vi "Get Station Number.vi"(8 "error in (no error)":errorcluster, 11 "UI Data in":T1) -> (0 "error out (no error)":errorcluster, 3 "UI Data out":T1)   [LabVIEW 2016]
uses:
  controls/GLDL UI Data.ctl
  controls/Disconnect Control.ctl
  controls/Download Control.ctl
  controls/Exit Control.ctl
  controls/Date Control.ctl
  controls/Save Path Control.ctl
  controls/COM Port Control.ctl
  controls/IP Phone Number Control.ctl
  controls/Connected Indicator.ctl
  controls/Output Indicator.ctl
  Message Queue/All Message Queues.ctl
  Message Queue/Message Cluster.ctl
  Message Queue/GLDL Message Queue.lvlib
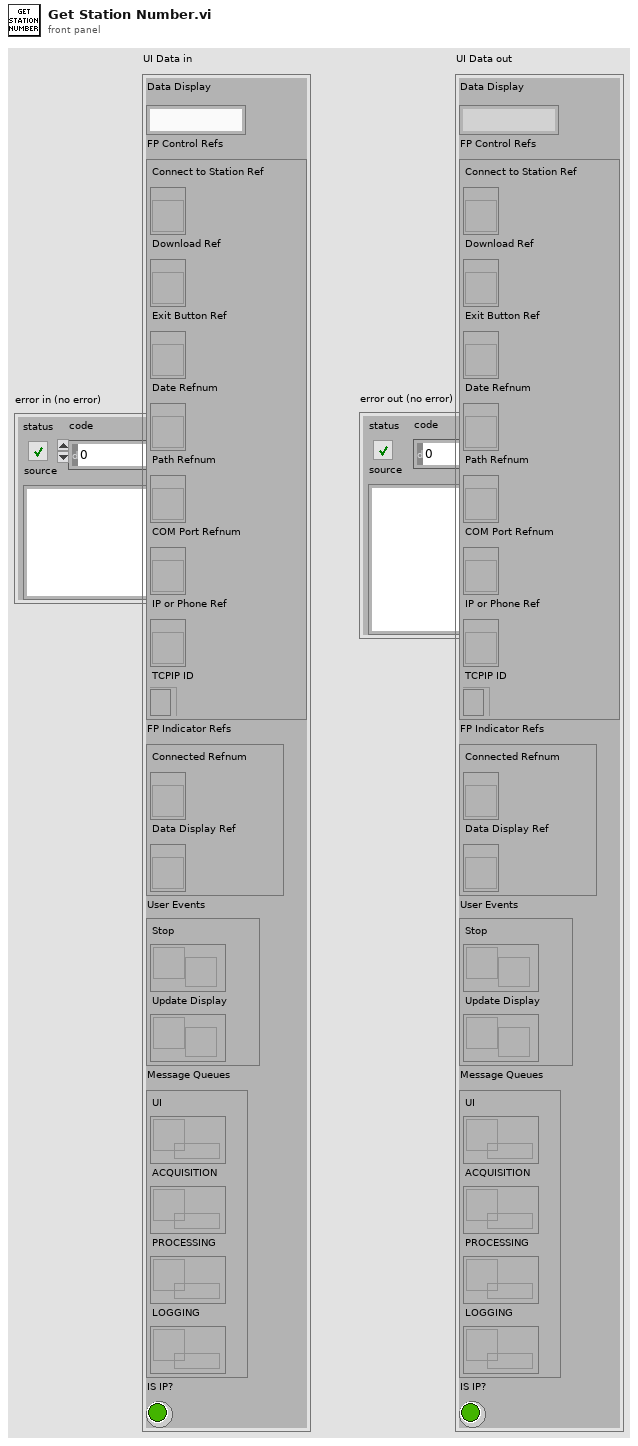
[diagram p1: front panel]
types:
  T1 = typedef "GLDL UI Data.ctl" = cluster{"Data Display":string, "FP Control Refs":cluster{"Connect to Station Ref":refnum<vi>, "Download Ref":refnum<vi>, "Exit Button Ref":refnum<vi>, "Date Refnum":refnum<vi>, "Path Refnum":refnum<vi>, "COM Port Refnum":refnum<vi>, "IP or Phone Ref":refnum<vi>, "TCPIP ID":refnum<k5>}, "FP Indicator Refs":cluster{"Connected Refnum":refnum<vi>, "Data Display Ref":refnum<vi>}, "User Events":cluster{"Stop":refnum<user-event>, "Update Display":refnum<user-event>}, "Message Queues":T2, "IS IP?":bool}
  T2 = typedef "GLDL Message Queue.lvlib/All Message Queues.ctl" = cluster{"UI":refnum<queue>, "ACQUISITION":refnum<queue>, "PROCESSING":refnum<queue>, "LOGGING":refnum<queue>}
  T3 = enum16{"Standard", "Buffered", "CRLF", "Immediate"}
  T4 = typedef "COM Port Control.ctl" = refnum<visa-resource-name>
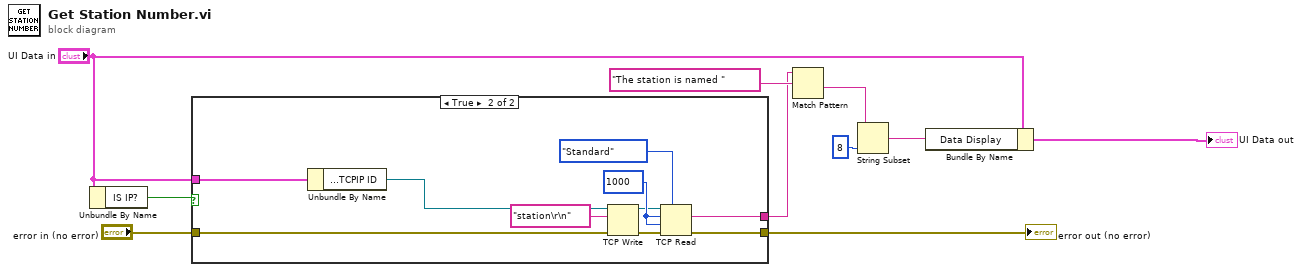
[diagram p0: block diagram]
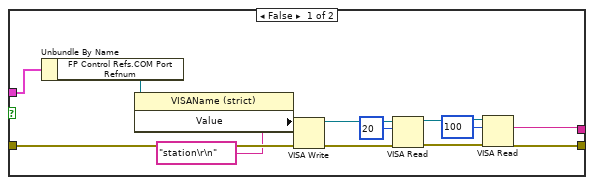
[diagram p2: hidden frame]
diagram:
  n1 = Unbundle By Name("UI Data in") -> ("IS IP?"=w3:bool)
  n2 = case shown="True" w3 {
    tunnel: "error in (no error)" -> [w20 w28]
    tunnel: [w12 w27] -> w8
    tunnel: [w11 w26] -> w4
    tunnel: "UI Data in" -> [w23 w24]
    frame False {
      n3 = Unbundle By Name(w23) -> ("FP Control Refs.COM Port Refnum"=w22:refnum<vi>)
      n4 = property class="VISAName (strict)"(reference=w22) -> ("Value"=w21:T4)  [unwired: 1 in, 2 out]
      n5 = VISA Write(VISA resource name=w21, write buffer="station\r\n", error in (no error)=w20) -> (VISA resource name out=w17:T4, error out=w18:errorcluster)  [unwired: 1 out]
      n6 = VISA Read(VISA resource name=w17, byte count=u32 20, error in (no error)=w18) -> (VISA resource name out=w14:T4, error out=w13:errorcluster)  [unwired: 2 out]
      n7 = VISA Read(VISA resource name=w14, byte count=u32 100, error in (no error)=w13) -> (read buffer=w12:string, error out=w11:errorcluster)  [unwired: 2 out]
    }
    frame True {
      w33 = 1000 ("timeout ms (25000)")
      n8 = Unbundle By Name(w24) -> ("FP Control Refs.TCPIP ID"=w25:refnum<k5>)
      n9 = TCP Write(connection ID=w25, data in="station\r\n", error in (no error)=w28) -> (connection ID out=w31:refnum<k5>, error out=w30:errorcluster)  [unwired: 1 in, 1 out]
      n10 = TCP Read(connection ID=w31, bytes to read=w33, error in (no error)=w30, 7:T3."Standard" ("mode (standard)"), 9:w33) -> (data out=w27:string, error out=w26:errorcluster)  [unwired: 1 out]
    }
  }
  "error out (no error)" <- w4
  n11 = Match Pattern(string=w8, regular expression="The station is named ") -> (after substring=w7:string)  [unwired: 1 in, 3 out]
  n12 = String Subset(string=w7, length (rest)=8 ("length (rest)")) -> (substring=w6:string)  [unwired: 1 in]
  n13 = Bundle By Name(cluster="UI Data in", "Data Display"=w6) -> (→"UI Data out":T1)
